vi "TABSpeed.vi"(3 "Boxcar Average":dbl[](array[numeric]), 4 "Current Position":T1, 5 "Old Position":T3) -> (0 "New Speed of Boat\nin Pixels/Sec":dbl, 1 "Boxcar Average Out":dbl[](array[numeric]), 2 "New Position":T2)   [LabVIEW 2014]
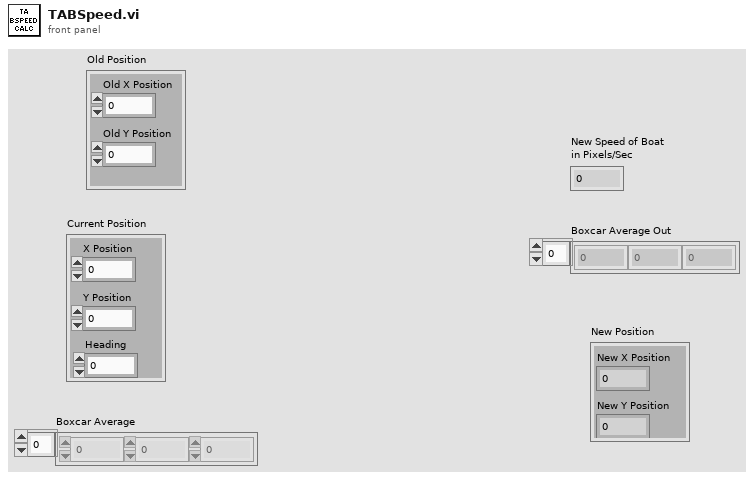
[diagram p1: front panel]
types:
  T1 = cluster{"X Position":i32, "Y Position":i32, "Heading":i32}
  T2 = cluster{"New X Position":i32, "New Y Position":i32}
  T3 = cluster{"Old X Position":i32, "Old Y Position":i32}
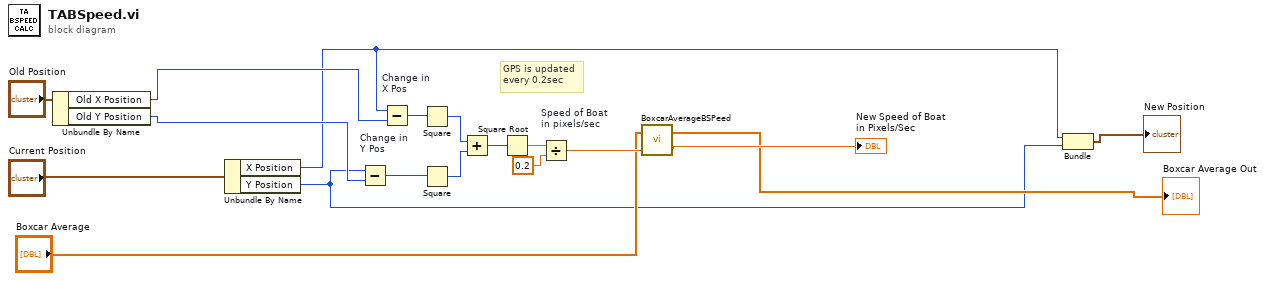
[diagram p0: block diagram]
diagram:
  # "GPS is updated\nevery 0.2sec"
  n1 = Unbundle By Name("Old Position") -> ("Old X Position"=w9:i32, "Old Y Position"=w10:i32)
  n2 = Unbundle By Name("Current Position") -> ("X Position"=w8:i32, "Y Position"=w1:i32)
  n3 = Subtract "Change in \nY Pos"(x=w1, y=w10) -> (x-y=w17:i32)
  n4 = Subtract "Change in \nX Pos"(x=w8, y=w9) -> (x-y=w18:i32)
  n5 = Square(x=w18) -> (x^2=w15:i32)
  n6 = Square(x=w17) -> (x^2=w16:i32)
  n7 = Add(x=w15, y=w16) -> (x+y=w14:i32)
  n8 = Square Root(x=w14) -> (sqrt(x)=w13:dbl)
  n9 = Divide "Speed of Boat\nin pixels/sec"(x=w13, y=0.2) -> (x/y=w6:dbl)
  n10 = call "BoxcarAverageBSPeed.vi"("Boat Speed In"=w6, "Box Car Average In"="Boxcar Average") -> ("Boat Speed Out"=→"New Speed of Boat\nin Pixels/Sec":dbl, "Box Car Average Out"=→"Boxcar Average Out":dbl[])
  n11 = Bundle("X Position"=w8, "Y Position"=w1) -> (→"New Position":cluster{"X Position":i32, "Y Position":i32})  [unwired: 1 in]
